vi "Write UniqueIDs.vi"(10 "UniqueIDs":string[](array[string]), 11 "Parallel in":refnum<class "Parallel.lvclass">) -> (3 "Parallel out":refnum<class "Parallel.lvclass">)   [LabVIEW 2019, in "Test Executive.lvlib" / "Parallel.lvclass"]
uses:
  <vilib>/gpm_packages/@cs/test-executive/Source/Test Executive/Parallel/Parallel.lvclass
  <vilib>/gpm_packages/@cs/test-executive/Source/Test Executive/Parallel/Parallel.lvclass/Parallel.ctl
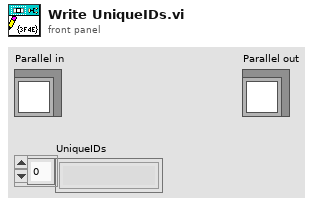
[diagram p1: front panel]
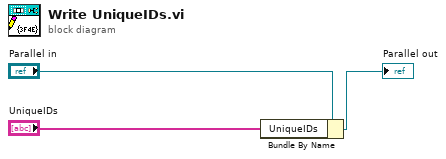
[diagram p0: block diagram]
diagram:
  n1 = Bundle By Name(cluster="Parallel in", "UniqueIDs"="UniqueIDs") -> (→"Parallel out":refnum<class "Parallel.lvclass">)
